vi "Edita_lista.vi"() -> (2 "lista Auxiliar":string[][](table))   [LabVIEW 2012]
panel:
  out "Lista Antiga":string[][](array[string])
  in  "lista":string[][](table)
  in  "Cancel":bool
  in  "SAVE":bool
  in  "Multicolumn Listbox":i32[](listbox)
  # "Edit the Item and soon after press SAVE or Cancel"
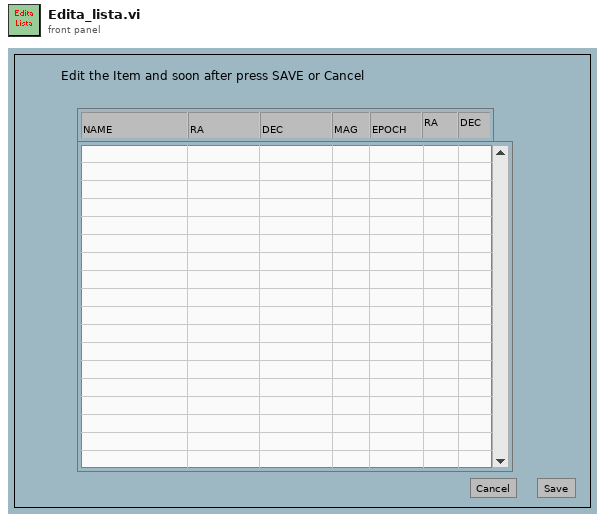
[diagram p1: front panel]
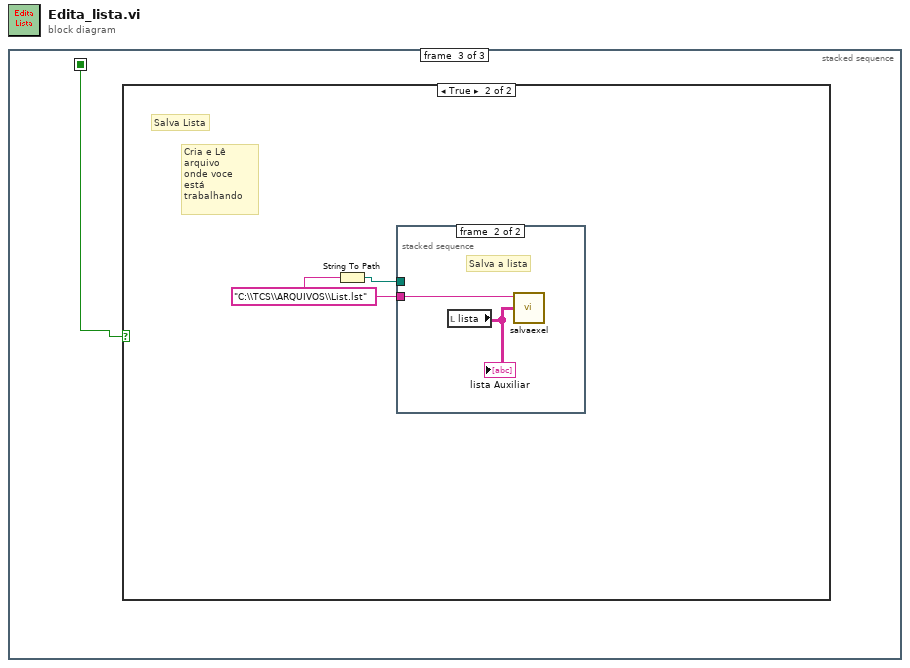
[diagram p0: block diagram]
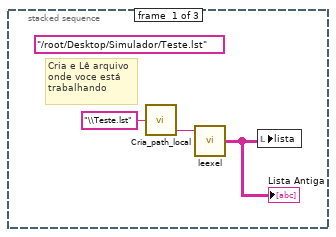
[diagram p2: hidden frame]
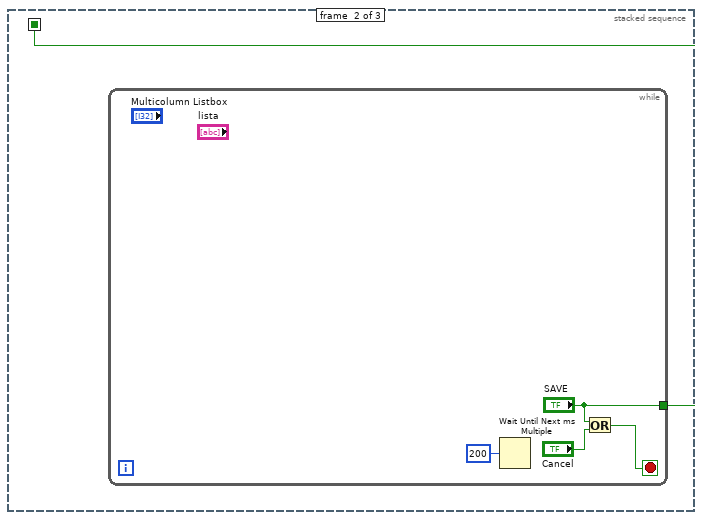
[diagram p3: hidden frame]
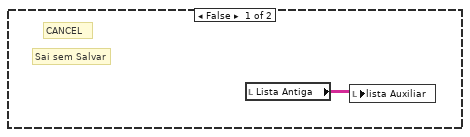
[diagram p4: hidden frame]
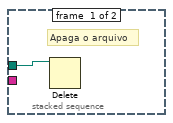
[diagram p5: hidden frame]
diagram:
  n1 = stacked-sequence {
    seq-local: [_ w4 _] -> [_ _ w9]
    frame #0 {
      (unwired) "/root/Desktop/Simulador/Teste.lst" ("caminho final")
      # "Cria e Lê arquivo\nonde voce está\ntrabalhando"
      n2 = call "Cria_path_local.vi"("caminho final"="\\Teste.lst") -> ("Saida Path string"=w2:string)  [unwired: 3 in, 1 out]
      n3 = call "leexel.vi"("path"=w2) -> ("array 5"=w3:string[][])  [unwired: 4 in]
      "Lista Antiga" <- w3
      n4 = local write "lista"(w3) -> ()
    }
    frame #1 {
      n5 = while {
        tunnel: ["SAVE"] -> w4
        stop <- w7 stop-if-true
        n6 = Wait Until Next ms Multiple(millisecond multiple=u32 200) -> ()  [unwired: 1 out]
        n7 = Or(x="SAVE", y="Cancel") -> (x .or. y?=w7:bool)
      }
    }
    frame #2 {
      n8 = case shown="True" w9 {
        frame False {
          # "CANCEL"
          # "Sai sem Salvar"
          n9 = local read "Lista Antiga"() -> (w10:string[][])
          n10 = local write "lista Auxiliar"(w10) -> ()
        }
        frame True {
          w12 = "C:\\TCS\\ARQUIVOS\\List.lst"
          # "Cria e Lê arquivo\nonde voce está\ntrabalhando"
          # "Salva Lista"
          n11 = String To Path(string=w12) -> (path=w11:path)
          n12 = stacked-sequence {
            tunnel: w11 -> [w13 _]
            tunnel: w12 -> [_ w15]
            frame #0 {
              # "Apaga o arquivo"
              n13 = Delete(path (use dialog)=w13) -> ()  [unwired: 4 in, 3 out]
            }
            frame #1 {
              # "Salva a lista"
              n14 = local read "lista"() -> (w14:string[][])
              "lista Auxiliar" <- w14
              n15 = call "salvaexel.vi"("appended array"=w14, "file name p/ exell"=w15) -> ()  [unwired: 1 in, 1 out]
            }
          }
        }
      }
    }
  }
